vi "DepthProfile_Setup.vi"(7 "RepRate (Hz)":dbl=1000.0 min=0.0, 10 "Start Position":dbl[](array[numeric]) min=0.0 max=34.0) -> (1 "Depth Profile Params.":T2={"SamplingPos."=[], "z-depth (ms)"=0, "Idle(ms)"=0, "HighSpeed"=0.0, "RepRate (Hz)"=1000.0} {"RepRate (Hz)" min=0.0}, 2 "Canceled":bool, 3 "Meander_Params.":T1, 5 "SaveRaw":bool)   [LabVIEW 2013]
uses:
  DepthProfilingParams.ctl
  Files/BinaryHeader.ctl
panel:
  in  "Save Raw File?":bool
  in  "HighSpeed":dbl=10.0 min=0.0
  in  "Interval (ms)":u32 caption="Shots interval (ms)"
  out "Estimated Time":dbl caption="Estimated Time (min)" min=0.0 max=34.0
  in  "Z-Depth":u32=100
  in  "Apply":bool
  in  "Cancel":bool
  in  "Run":bool
  out "XY Graph":cluster{dbl, "X StepWidth":dbl, dbl}[](graph)
  out "2ndAxialSize":dbl caption="Y Size (mm)" min=0.0 max=34.0
  out "1stAxialSize":dbl caption="X Size (mm)" min=0.0 max=34.0
  in  "2ndAxialSteps":i32=10 caption="Y Steps" min=0
  in  "1stAxialSteps":i32=10 caption="XSteps" min=0
  in  "StepWidth":dbl=0.2 min=0.0
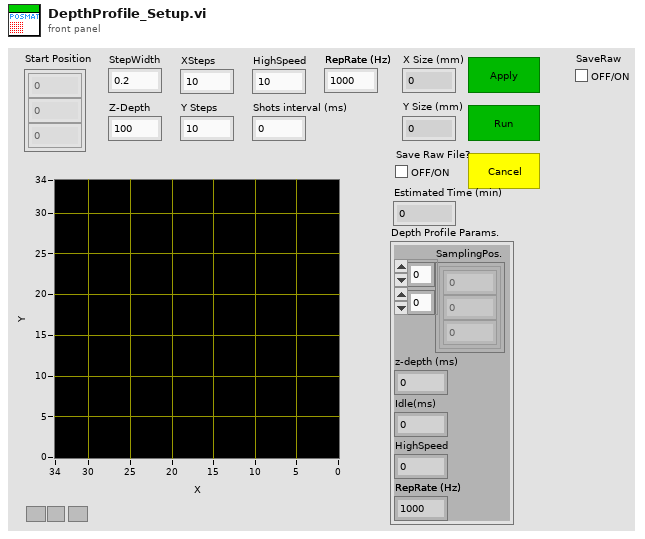
[diagram p1: front panel]
types:
  T1 = typedef "BinaryHeader.ctl" = cluster{"Start Position":dbl[], "StepWidth":dbl[], "Dimension":i32[], "SpecLength":i32}
  T2 = typedef "DepthProfilingParams.ctl" = cluster{"SamplingPos.":cluster{"x":dbl, "y":dbl, "z":dbl}[][], "z-depth (ms)":u32, "Idle(ms)":u32, "HighSpeed":dbl, "RepRate (Hz)":dbl}
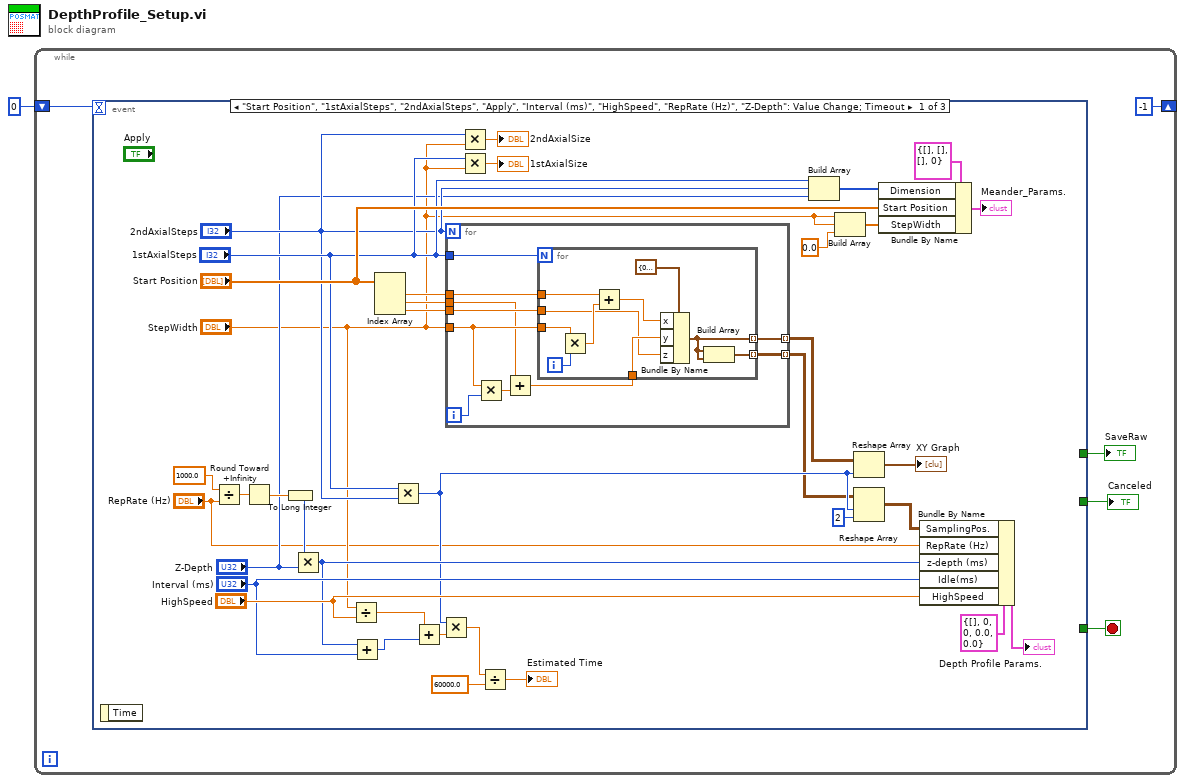
[diagram p0: block diagram]
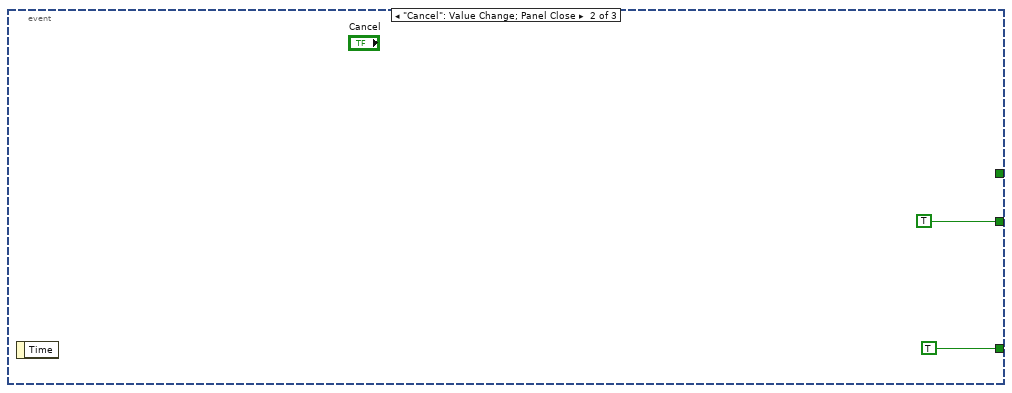
[diagram p2: hidden frame]
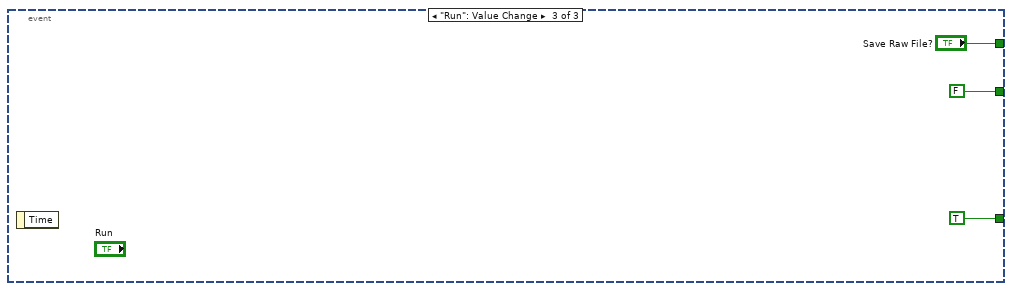
[diagram p3: hidden frame]
diagram:
  n1 = while {
    shift-right: [-1] -> _
    shift-left: 0 -> [w4]
    stop <- w6 stop-if-true
    n2 = event shown="[0] \"Start Position\", \"1stAxialSteps\", \"2ndAxialSteps\", \"Apply\", \"Interval (ms)\", \"HighSpeed\", \"RepRate (Hz)\", \"Z-Depth\": Value Change;  Timeout" {
      selector: _ -> [_ _ _]
      dyn-events: _ -> [_ _ _]
      timeout: w4 -> [_ _ _]
      tunnel: [_ TRUE TRUE] -> w6
      tunnel: [_ TRUE ("Canceled") FALSE ("Canceled")] -> w5
      tunnel: [_ _ "Save Raw File?"] -> w2
      event "Start Position", "1stAxialSteps", "2ndAxialSteps", "Apply", "Interval (ms)", "HighSpeed", "RepRate (Hz)", "Z-Depth": Value Change; Timeout {
        n3 = event-data() -> ()  [unwired: 1 in, 1 out]
        n4 = Divide(x=1000.0 ("value"), y="RepRate (Hz)") -> (x/y=w10:dbl)
        n5 = Round Toward +Infinity(x=w10) -> (ceil(x): smallest int >= x=w19:dbl)
        n6 = To Long Integer(number=w19) -> (32bit integer=w18:i32)
        n7 = Multiply(x=w18, y="Z-Depth") -> (x*y=w20:u32)
        n8 = Divide(x="StepWidth", y="HighSpeed") -> (x/y=w23:dbl)
        n9 = Add(x=w20, y="Interval (ms)") -> (x+y=w22:u32)
        n10 = Index Array(array="Start Position") -> (element #1=w43:dbl, element #2=w37:dbl, element #3=w38:dbl)  [unwired: 3 in]
        n11 = Multiply(x="1stAxialSteps", y="2ndAxialSteps") -> (x*y=w16:i32)
        n12 = Add(x=w23, y=w22) -> (x+y=w40:dbl)
        n13 = Multiply(x=w16, y=w40) -> (x*y=w32:dbl)
        n14 = for {
          N: "2ndAxialSteps" -> [_]
          tunnel: w38 -> [w46]
          tunnel: "StepWidth" -> [w48]
          tunnel: [w50] -> w15 mode=indexing
          tunnel: w37 -> [w45]
          tunnel: "1stAxialSteps" -> [w47]
          tunnel: w43 -> [w49]
          tunnel: [w44] -> w13 mode=indexing
          i -> [w53]
          n15 = Multiply(x=w48, y=w53) -> (x*y=w52:dbl)
          n16 = Add(x=w45, y=w52) -> (x+y=w51:dbl)
          n17 = for {
            N: w47 -> [_]
            tunnel: w48 -> [w61]
            tunnel: w49 -> [w59]
            tunnel: w51 -> [w58]
            tunnel: [w55] -> w50 mode=indexing
            tunnel: w46 -> [w57]
            tunnel: [w54] -> w44 mode=indexing
            i -> [w62]
            n18 = Multiply(x=w61, y=w62) -> (x*y=w63:dbl)
            n19 = Add(x=w59, y=w63) -> (x+y=w60:dbl)
            n20 = Bundle By Name(cluster=cluster{"x":dbl, "y":dbl, "z":dbl} {"x"=0.0, "y"=0.0, "z"=0.0}, "x"=w60, "y"=w58, "z"=w57) -> (w55:cluster{"x":dbl, "y":dbl, "z":dbl})
            n21 = Build Array(w55, w55) -> (w54:cluster{"x":dbl, "y":dbl, "z":dbl}[])
          }
        }
        n22 = Multiply(x="2ndAxialSteps", y="StepWidth") -> (x*y=→"2ndAxialSize":dbl)
        n23 = Multiply(x="1stAxialSteps", y="StepWidth") -> (x*y=→"1stAxialSize":dbl)
        n24 = Divide(x=w32, y=60000.0) -> (x/y=→"Estimated Time":dbl)
        n25 = Build Array("1stAxialSteps", "2ndAxialSteps", "Z-Depth") -> (w30:u32[])
        n26 = Build Array("StepWidth", "StepWidth", 0.0 ("element")) -> (w29:dbl[])
        n27 = Reshape Array(w15, w16) -> (→"XY Graph":cluster{"x":dbl, "y":dbl, "z":dbl}[])
        n28 = Reshape Array(w13, w16, 2 ("dimension size")) -> (w12:cluster{"x":dbl, "y":dbl, "z":dbl}[][])
        n29 = Bundle By Name(cluster=T1 {"Start Position"=[], "StepWidth"=[], "Dimension"=[], "SpecLength"=0} ("File Header"), "Dimension"=w30, "Start Position"="Start Position", "StepWidth"=w29) -> (→"Meander_Params.":T1)
        n30 = Bundle By Name(cluster=T2 {"SamplingPos."=[], "z-depth (ms)"=0, "Idle(ms)"=0, "HighSpeed"=0.0, "RepRate (Hz)"=0.0} ("Depth Profile Params. 2"), "SamplingPos."=w12, "RepRate (Hz)"="RepRate (Hz)", "z-depth (ms)"=w20, "Idle(ms)"="Interval (ms)", "HighSpeed"="HighSpeed") -> (→"Depth Profile Params.":T2)
      }
      event "Cancel": Value Change; Panel Close {
        n31 = event-data() -> ()  [unwired: 1 in, 1 out]
      }
      event "Run": Value Change {
        n32 = event-data() -> ()  [unwired: 1 in, 1 out]
      }
    }
    "Canceled" <- w5
    "SaveRaw" <- w2
  }
